vi "Format Structure Table.vi"(11 "Structure Tree Array in":T1[](array[typedef])) -> (3 "String":string)   [LabVIEW 2023, in "VIDoc Printer - Confluence.lvlib" / "VIDoc Printer - Confluence.lvclass"]
uses:
  VIDoc Printer - Confluence.lvclass
  Parsing/SubVIs/Structure Reporter/Tree Cluster.ctl
  VIDoc Printer - Confluence.lvclass/VIDoc Printer - Confluence.ctl
  Confluence Formatting/Confluence Formatting.lvlib
  <userlib>/_PetranWay/LabVIEW Confluence API/Source/PetranWay_Confluence API.lvlib
  Parsing/SubVIs/Structure Reporter/Structure Reporter.lvlib
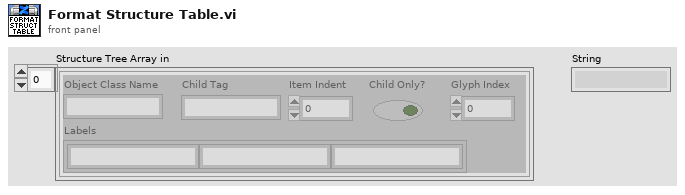
[diagram p1: front panel]
types:
  T1 = typedef "VIDoc Parsing.lvlib/Structure Reporter.lvlib/Tree Cluster.ctl" = cluster{"Object Class Name":string, "Labels":string[], "Child Tag":string, "Item Indent":i32, "Child Only?":bool, "Glyph Index":i32}
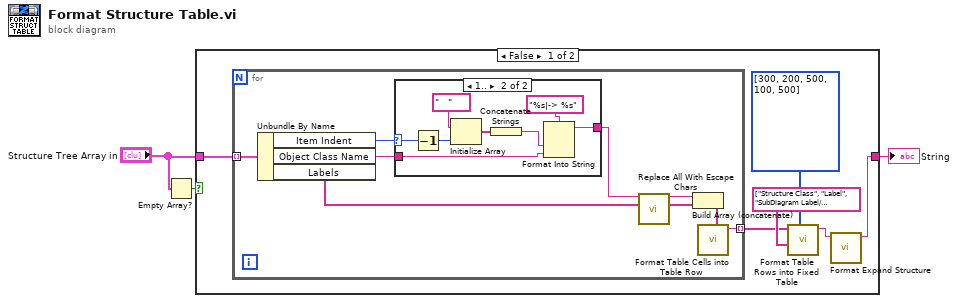
[diagram p0: block diagram]
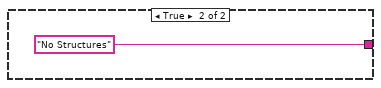
[diagram p3: hidden frame]
diagram:
  n1 = Empty Array?(array="Structure Tree Array in") -> (empty?=w1:bool)
  n2 = case shown="False" w1 {
    tunnel: "Structure Tree Array in" -> [w5 _]
    tunnel: [w9 "No Structures"] -> w3
    frame False {
      n3 = for {
        tunnel: [w17] -> w6 mode=indexing
        tunnel: w5 -> [w16] mode=indexing
        n4 = Unbundle By Name(w16) -> ("Item Indent"=w15:i32, "Object Class Name"=w14:string, "Labels"=w12:string[])
        n5 = case shown="1.." w15 {
          selector: w15 -> [_ w26]
          tunnel: w14 -> [w18 w24]
          tunnel: [w18 w23] -> w13
          frame ..0 {
          }
          frame 1.. {
            n6 = Decrement(x=w26) -> (x-1=w19:i32)
            n7 = Initialize Array("   ", w19) -> (w22:string[])
            n8 = Concatenate Strings(w22) -> (w21:string)
            n9 = Format Into String(format string="%s|-> %s", w21, w24) -> (resulting string=w23:string)  [unwired: 2 in, 1 out]
          }
        }
        n10 = call <userlib>:"Replace All With Escape Chars.vi"("Raw String"=w13) -> ("With Substitued Escape Characters"=w10:string)  [unwired: 13 in, 1 out]
        n11 = Build Array (concatenate)(w10, w12) -> (w11:string[])
        n12 = call "Format Table Cells into Table Row.vi"("Table Cells"=w11) -> ("Table Row Text"=w17:string)  [unwired: 10 in]
      }
      n13 = call "Format Table Rows into Fixed Table.vi"("Column Pixel Widths"=i16[] [300, 200, 500, 100, 500], "Table Headers"=string[] ["Structure Class", "Label", "SubDiagram Label/Description", "Frame I", "Frame Condition"], "Table Rows"=w6) -> ("Table Text"=w8:string)  [unwired: 8 in]
      n14 = call "Format Expand Structure.vi"("Content"=w8) -> ("Expand String"=w9:string)  [unwired: 9 in, 1 out]
    }
    frame True {
    }
  }
  "String" <- w3
